vi "Rapidox read MAX FPGA.vi"() -> (2 "Output":u8[](array[numeric]))   [LabVIEW 2011]
uses:
  <vilib>/rvi/eio/common/nirviEmuTemplateMethod_errors.vi
  <vilib>/eio/EIOMethodNode/EIOMethodNode.xnode
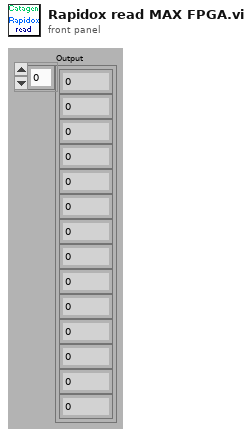
[diagram p1: front panel]
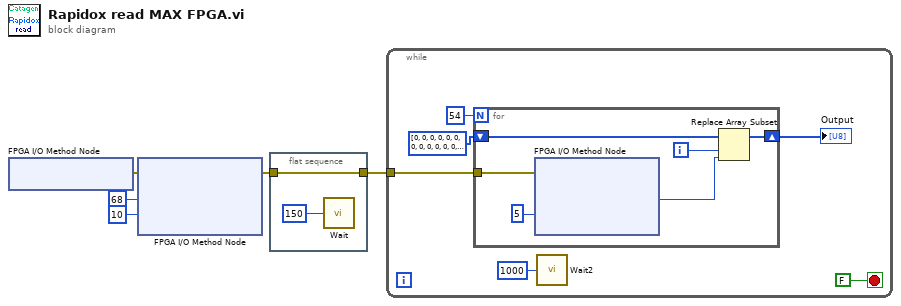
[diagram p0: block diagram]
diagram:
  n1 = xnode "FPGA I/O Method Node"() -> ("error out"=w3:errorcluster)  [unwired: 2 in, 1 out]
  n2 = xnode "FPGA I/O Method Node"("error in"=w3, "Data"=u8 68, "Timeout (ms)"=10) -> ("error out"=w2:errorcluster)  [unwired: 1 in, 2 out]
  n3 = flat-sequence {
    tunnel: w2 -> [w7]
    tunnel: [w7] -> w1
    frame #0 {
      n4 = call "Wait"("Count(mSec)"=u32 150) -> ()  [unwired: 1 out]
    }
  }
  n5 = while {
    tunnel: w1 -> [w10]
    stop <- FALSE stop-if-true
    n6 = for {
      N: 54 -> [_]
      tunnel: w10 -> [w19]
      shift-right: [w15] -> w12
      shift-left: u8[] [0, 0, 0, 0, 0, 0, 0, 0, 0, 0, 0, 0, 0, 0, 0, 0, 0, 0, 0, 0, 0, 0, 0, 0, 0, 0, 0, 0, 0, 0, 0, 0, 0, 0, 0, 0, 0, 0, 0, 0, 0, 0, 0, 0, 0, 0, 0, 0, 0, 0, 0, 0, 0, 0] -> [w17]
      i -> [w14]
      n7 = xnode "FPGA I/O Method Node"("error in"=w19, "Timeout (ms)"=5) -> ("Data"=w16:u8)  [unwired: 1 in, 3 out]
      n8 = Replace Array Subset(array=w17, new element=w16, index=w14) -> (w15:u8[])
    }
    "Output" <- w12
    n9 = call "Wait2"("Count(mSec)"=u32 1000) -> ()  [unwired: 1 out]
  }
